vi "Server.vi"   [LabVIEW 2015]
uses:
  Data/Nicholas Data.lvclass
  CRD/nCRD.lvclass
  PAS/nPAS.lvclass
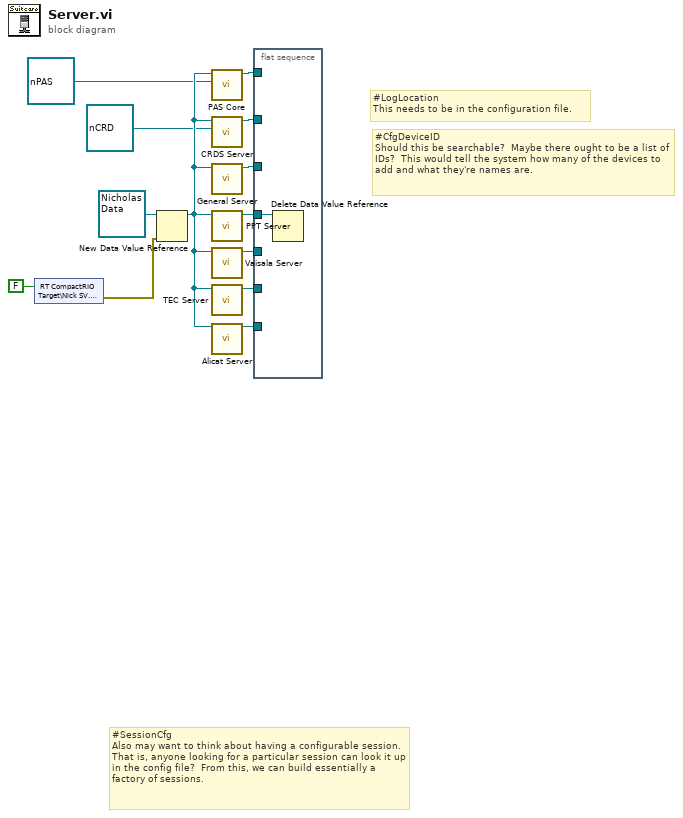
[diagram p0: block diagram]
diagram:
  # "#SessionCfg\nAlso may want to think about having a configurable session.  That is, anyone looking for a particular session can look it up in the config file?  From this, we can build essentially a factory of sessions."
  # "#CfgDeviceID\nShould this be searchable?  Maybe there ought to be a list of IDs?  This would tell the system how many of the devices to add and what they're names are."
  # "#LogLocation\nThis needs to be in the configuration file."
  n1 = shared-variable "RT CompactRIO Target\\Nick SV.lvlib\\Stop"(FALSE ("Stop")) -> (error out=w3:errorcluster)  [unwired: 1 in]
  n2 = New Data Value Reference(data value=refnum<class "Nicholas Data.lvclass"> refnum ("Nicholas Data.lvclass"), error in=w3) -> (data value reference=w5:refnum<data-value>)  [unwired: 1 out]
  n3 = call "PAS Core.vi"("nPAS In"=refnum<class "nPAS.lvclass"> refnum ("nPAS"), "DVR In"=w5) -> ("nPAS out"=w11:refnum<class "nPAS.lvclass">)  [unwired: 9 in]
  n4 = call "CRDS Server.vi"("nCRD in"=refnum<class "nCRD.lvclass"> refnum ("nCRD"), "DVR In"=w5) -> ("nCRD out"=w12:refnum<class "nCRD.lvclass">)  [unwired: 9 in]
  n5 = call "General Server.vi"("DVR In"=w5) -> ("FPGA Session out"=w10:refnum<class "FPGA Session.lvclass">)  [unwired: 10 in]
  n6 = call "PPT Server.vi"("DVR In"=w5) -> ("DVR Out"=w8:refnum<data-value>)  [unwired: 10 in]
  n7 = call "Vaisala Server.vi"("DVR In"=w5) -> ("DVR Out"=w7:refnum<data-value>)  [unwired: 10 in]
  n8 = call "TEC Server.vi"("DVR In"=w5) -> ("DVR Out"=w6:refnum<data-value>)  [unwired: 10 in]
  n9 = call "Alicat Server.vi"("DVR In"=w5) -> ("DVR out"=w9:refnum<data-value>)  [unwired: 18 in]
  n10 = flat-sequence {
    tunnel: w12 -> [_]
    tunnel: w11 -> [_]
    tunnel: w10 -> [_]
    tunnel: w9 -> [_]
    tunnel: w8 -> [w14]
    tunnel: w7 -> [_]
    tunnel: w6 -> [_]
    frame #0 {
      n11 = Delete Data Value Reference(data value reference=w14) -> ()  [unwired: 1 in, 2 out]
    }
  }
